vi "Write Generic.DeviceName.vi"(8 "error in (no error)":errorcluster, 10 "Generic.DeviceName":string, 11 "GenericCamera in":refnum<class "GenericCamera.lvclass">) -> (0 "error out":errorcluster, 3 "GenericCamera out":refnum<class "GenericCamera.lvclass">)   [LabVIEW 2013, in "GenericCamera.lvclass"]
uses:
  GenericCamera.lvclass
  GenericCamera.lvclass/GenericCamera.ctl
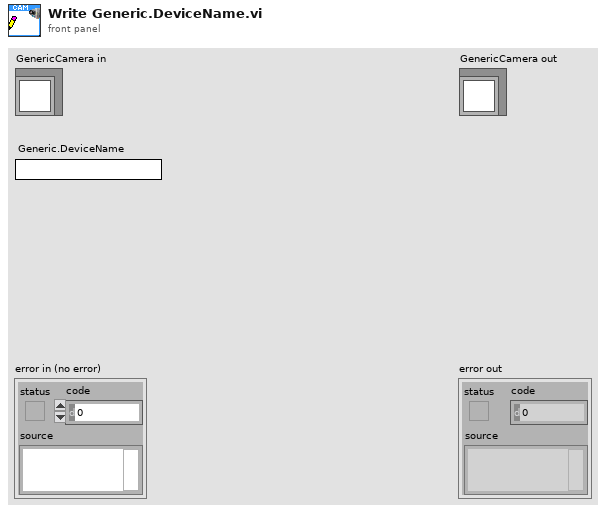
[diagram p1: front panel]
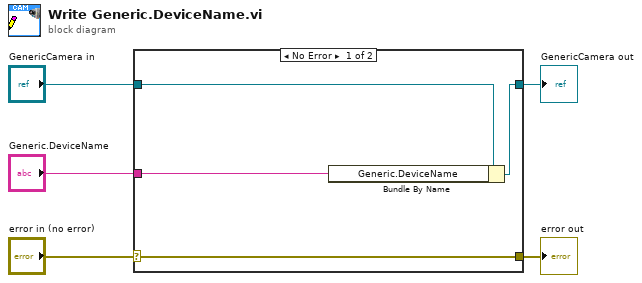
[diagram p0: block diagram]
diagram:
  n1 = case shown="No Error" "error in (no error)" {
    selector: "error in (no error)" -> [w9 w10]
    tunnel: [w9 w10] -> w4
    tunnel: [w7 w11] -> w2
    tunnel: "GenericCamera in" -> [w8 w11]
    tunnel: "Generic.DeviceName" -> [w6 _]
    frame No Error {
      n2 = Bundle By Name(cluster=w8, "Generic.DeviceName"=w6) -> (w7:refnum<class "GenericCamera.lvclass">)
    }
    frame Error {
    }
  }
  "error out" <- w4
  "GenericCamera out" <- w2
